vi "QuickOpen.vi"(11 "reference":refnum<vi>) -> ()   [LabVIEW 2020]
uses:
  <vilib>/regexp/Match Regular Expression.xnode
panel:
  in  "Search":string
  in  "Listbox":i32(listbox)
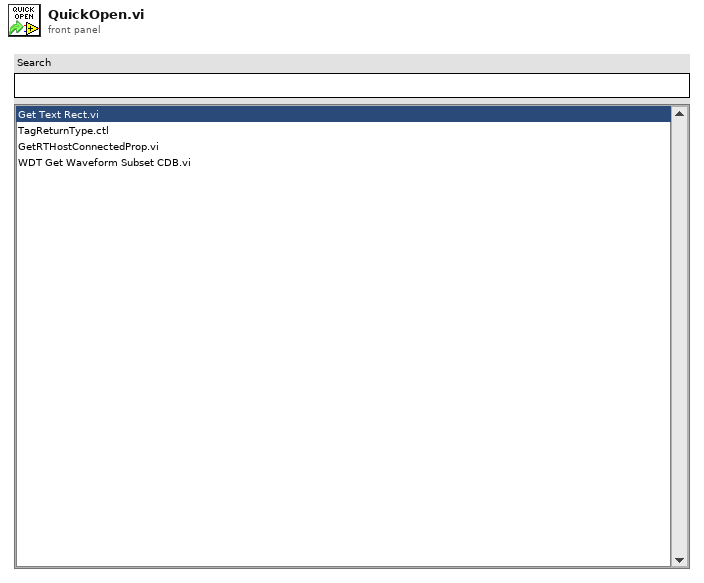
[diagram p1: front panel]
types:
  T1 = enum32{"Invalid", "Standard", "Closed", "Hidden", "Minimized", "Maximized"}
  T2 = typedef "eventvkey.ctl" = enum16{"ASCII", "Enter", "Return", "Shift", "Ctrl", "Alt", "Cmd", "Opt", "Caps", "NumLock", "Clear", "Break", "Up", "Down", "Left", "Right", "Insert", "Delete", "Home", "End", "PageUp", "PageDown", "Escape", "Help", "Pause", "ScrollLock", "F1", "F2", "F3", "F4", "F5", "F6", "F7", "F8", "F9", "F10", "F11", "F12", "F13", "F14", "F15", "F16", "F17", "F18", "F19", "F20", "F21", "F22", "F23", "F24", "Play", "VolumeUp", "VolumeDown", "Mute", "Two Byte Char"}
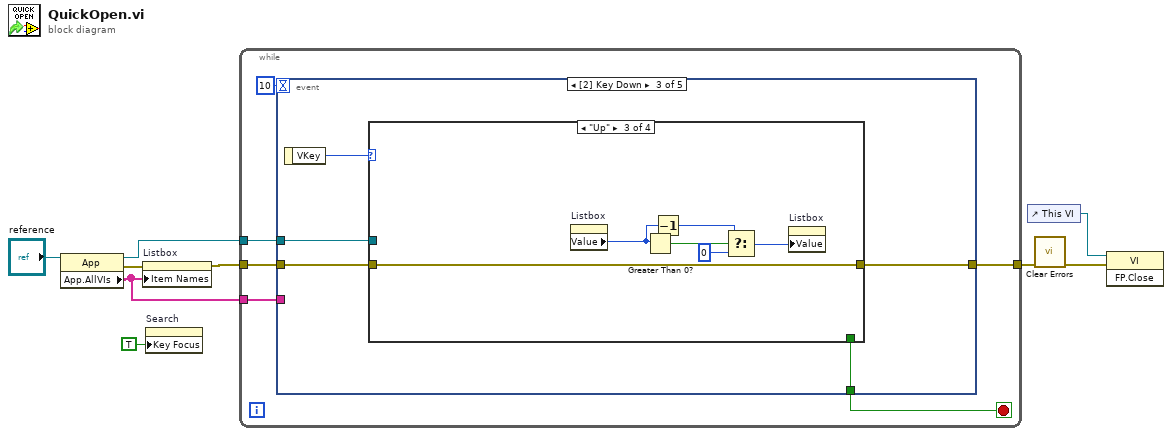
[diagram p0: block diagram]
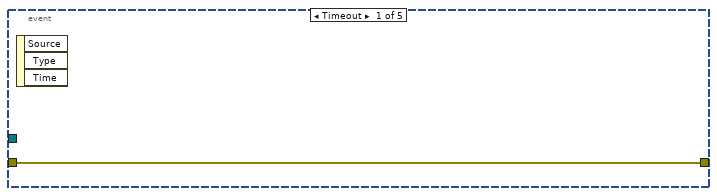
[diagram p2: hidden frame]
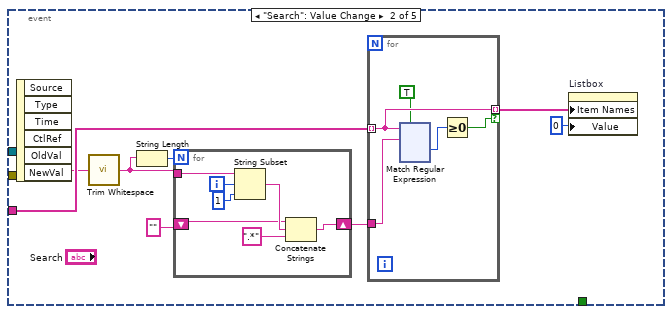
[diagram p3: hidden frame]
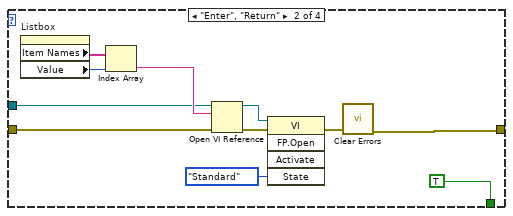
[diagram p5: hidden frame]
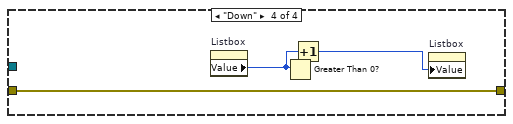
[diagram p6: hidden frame]
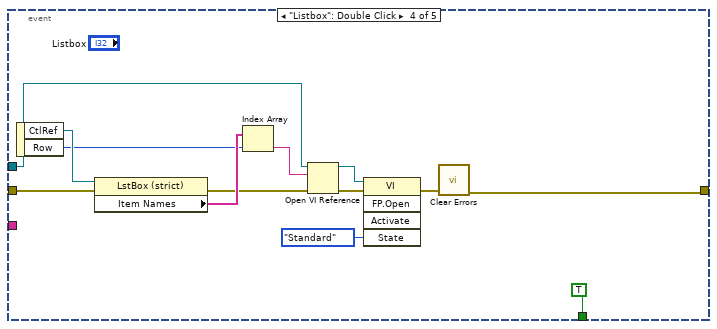
[diagram p7: hidden frame]
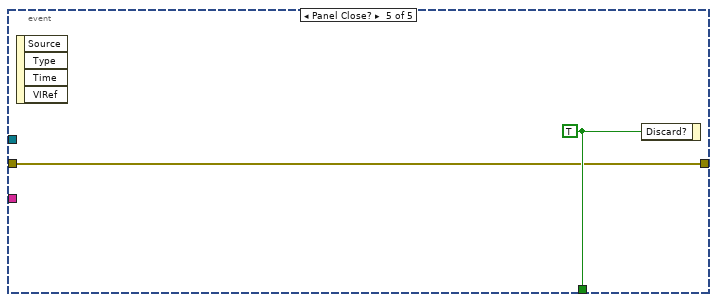
[diagram p8: hidden frame]
diagram:
  n1 = property class="App"(reference="reference") -> (reference out=w3:refnum<vi>, error out=w8:errorcluster, "App.AllVIs"=w9:string[])  [unwired: 1 in]
  n2 = property on="Listbox" class="LstBox (strict)"(error in=w8, "Item Names"=w9) -> (error out=w6:errorcluster)  [unwired: 1 in, 1 out]
  n3 = property on="Search" class="Str"("Key Focus"=TRUE) -> ()  [unwired: 2 in, 2 out]
  n4 = while {
    tunnel: w9 -> [w13]
    tunnel: w6 -> [w12]
    tunnel: [w11] -> w5
    tunnel: w3 -> [w10]
    stop <- w15 stop-if-true
    n5 = event shown="[2] Key Down" {
      selector: _ -> [_ _ _ _ _]
      dyn-events: _ -> [_ _ _ _ _]
      timeout: 10 -> [_ _ _ _ _]
      tunnel: [_ _ w154 TRUE w191] -> w15
      tunnel: w13 -> [_ w21 _ _ _]
      tunnel: w12 -> [w16 _ w153 w180 w190]
      tunnel: [w16 _ w152 w177 w190] -> w11
      tunnel: w10 -> [_ _ w151 w178 _]
      event Timeout {
        n6 = event-data() -> ()  [unwired: 1 in, 3 out]
      }
      event "Search": Value Change {
        n7 = event-data() -> ("NewVal"=w20:string)  [unwired: 1 in, 5 out]
        n8 = call <vilib>:"Trim Whitespace.vi"("string"=w20) -> ("trimmed string"=w18:string)  [unwired: 1 in]
        n9 = String Length(string=w18) -> (length=w24:i32)
        n10 = for {
          N: w24 -> [_]
          tunnel: w18 -> [w30]
          shift-right: [w29] -> w23
          shift-left: "" -> [w27]
          i -> [w31]
          n11 = String Subset(string=w30, offset (0)=w31, length (rest)=1 ("length (rest)")) -> (substring=w28:string)
          n12 = Concatenate Strings(w27, w28, ".*" ("string")) -> (w29:string)
        }
        n13 = for {
          tunnel: w21 -> [w33] mode=indexing
          tunnel: [w33] -> w19 mode=indexing if=w36
          tunnel: w23 -> [w35]
          n14 = xnode "Match Regular Expression"("input string"=w33, "regular expression"=w35, "ignore case? (F)"=TRUE) -> ("offset past match"=w34:i32)  [unwired: 3 in, 4 out]
          n15 = Greater Or Equal To 0?(x=w34) -> (x >= 0?=w36:bool)
        }
        n16 = property on="Listbox" class="LstBox (strict)"("Item Names"=w19, "Value"=0 ("Listbox")) -> ()  [unwired: 2 in, 2 out]
      }
      event Key Down {
        n17 = event-data() -> ("VKey"=w155:T2)  [unwired: 1 in]
        n18 = case shown="\"Up\"" w155 {
          tunnel: [_ TRUE _ _] -> w154
          tunnel: w153 -> [w156 w160 w168 w174]
          tunnel: [w156 w159 w168 w174] -> w152
          tunnel: w151 -> [_ w157 _ _]
          frame "ASCII", Default {
          }
          frame "Enter", "Return" {
            n19 = property on="Listbox" class="LstBox (strict)"() -> ("Item Names"=w165:string[], "Value"=w166:i32)  [unwired: 2 in, 2 out]
            n20 = Index Array(array=w165, index=w166) -> (element=w164:string)
            n21 = Open VI Reference(application reference (local)=w157, vi path=w164, error in (no error)=w160) -> (vi reference=w163:refnum<vi>, error out=w167:errorcluster)  [unwired: 3 in]
            n22 = invoke class="VI" method="FP.Open"(reference=w163, error in=w167, "State"=T1."Standard") -> (error out=w162:errorcluster)  [unwired: 2 in, 4 out]
            n23 = call <vilib>:"Clear Errors.vi"("error in (no error)"=w162) -> ("error out"=w159:errorcluster)  [unwired: 5 in, 1 out]
          }
          frame "Up" {
            n24 = property on="Listbox" class="LstBox (strict)"() -> ("Value"=w172:i32)  [unwired: 2 in, 2 out]
            n25 = Greater Than 0?(x=w172) -> (x > 0?=w173:bool)
            n26 = Decrement(x=w172) -> (x-1=w171:i32)
            n27 = Select(t=w171, s=w173, f=0) -> (s? t:f=w170:i32)
            n28 = property on="Listbox" class="LstBox (strict)"("Value"=w170) -> ()  [unwired: 2 in, 2 out]
          }
          frame "Down" {
            n29 = property on="Listbox" class="LstBox (strict)"() -> ("Value"=w176:i32)  [unwired: 2 in, 2 out]
            n30 = Greater Than 0?(x=w176) -> ()  [unwired: 1 out]
            n31 = Increment(x=w176) -> (x+1=w175:i32)
            n32 = property on="Listbox" class="LstBox (strict)"("Value"=w175) -> ()  [unwired: 2 in, 2 out]
          }
        }
      }
      event "Listbox": Double Click {
        n33 = event-data() -> ("CtlRef"=w182:refnum<vi>, "Row"=w181:i32)  [unwired: 1 in]
        n34 = property on="Property Node" class="LstBox (strict)"(reference=w182, error in=w180) -> (error out=w179:errorcluster, "Item Names"=w187:string[])  [unwired: 1 out]
        n35 = Index Array(array=w187, index=w181) -> (element=w186:string)
        n36 = Open VI Reference(application reference (local)=w178, vi path=w186, error in (no error)=w179) -> (vi reference=w185:refnum<vi>, error out=w188:errorcluster)  [unwired: 3 in]
        n37 = invoke class="VI" method="FP.Open"(reference=w185, error in=w188, "State"=T1."Standard") -> (error out=w184:errorcluster)  [unwired: 2 in, 4 out]
        n38 = call <vilib>:"Clear Errors.vi"("error in (no error)"=w184) -> ("error out"=w177:errorcluster)  [unwired: 5 in, 1 out]
      }
      event Panel Close? {
        w191 = TRUE ("Discard?")
        n39 = event-data() -> ()  [unwired: 1 in, 4 out]
        n40 = event-data("Discard?"=w191) -> ()  [unwired: 1 in, 1 out]
      }
    }
  }
  n41 = control-ref of="This VI"() -> (w2:refnum<vi>)
  n42 = call <vilib>:"Clear Errors.vi"("error in (no error)"=w5) -> ("error out"=w4:errorcluster)  [unwired: 5 in, 1 out]
  n43 = invoke class="VI" method="FP.Close"(reference=w2, error in=w4) -> ()  [unwired: 1 in, 3 out]
